vi "Return Value Manifester VI Path.vi"(11 "Manifestation Writer in":refnum<class "Manifestation Writer.lvclass">) -> (2 "Manifester VI Path":path, 3 "Manifestation Writer out":refnum<class "Manifestation Writer.lvclass">)   [LabVIEW 2013, in "Manifestation Writer.lvclass"]
doc: "Copyright (c) 2016 Sze Howe Koh\n\nThis Source Code Form is subject to the terms of the Mozilla Public License, v. 2.0. If a copy of the MPL was not distributed with this file, You can obtain one at http://mozilla.org/MPL/2.0/."
uses:
  Manifestation Writer.lvclass
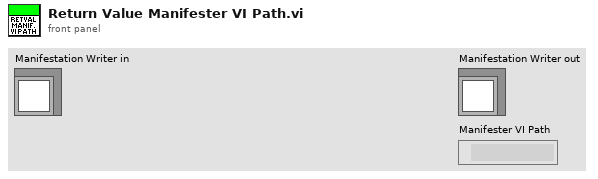
[diagram p1: front panel]
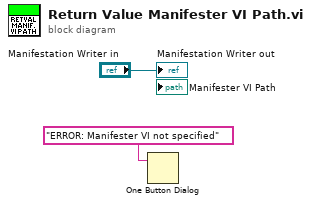
[diagram p0: block diagram]
diagram:
  n1 = One Button Dialog(message="ERROR: Manifester VI not specified") -> ()  [unwired: 1 in, 1 out]
  "Manifestation Writer out" <- "Manifestation Writer in"
